vi "Read Message queue.vi"(8 "error in (no error)":errorcluster, 11 "Parent Actor in":refnum<class "Parent Actor.lvclass">) -> (0 "error out":errorcluster, 2 "Message queue":refnum<queue>, 3 "Parent Actor out":refnum<class "Parent Actor.lvclass">)   [LabVIEW 2015, in "Parent Actor.lvclass"]
uses:
  Parent Actor.lvclass
  Parent Message/Parent Message.lvclass
  Parent Actor.lvclass/Parent Actor.ctl
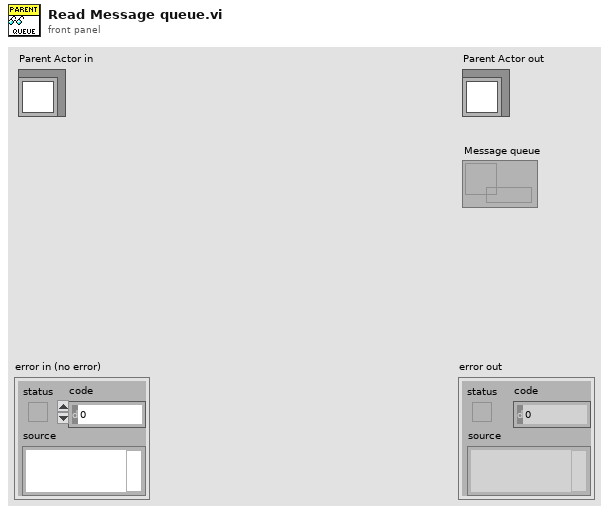
[diagram p1: front panel]
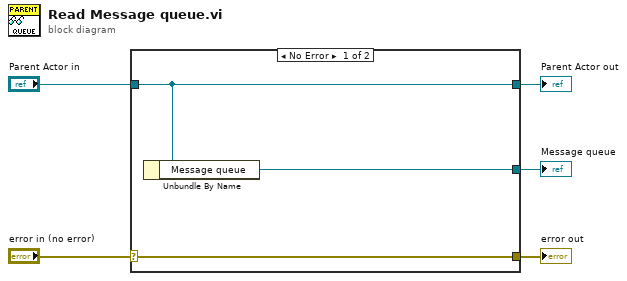
[diagram p0: block diagram]
diagram:
  n1 = case shown="No Error" "error in (no error)" {
    selector: "error in (no error)" -> [w8 w9]
    tunnel: [w8 w9] -> w4
    tunnel: [w7 w10] -> w2
    tunnel: "Parent Actor in" -> [w7 w10]
    tunnel: [w6 _] -> w1
    frame No Error {
      n2 = Unbundle By Name(w7) -> ("Message queue"=w6:refnum<queue>)
    }
    frame Error {
    }
  }
  "error out" <- w4
  "Parent Actor out" <- w2
  "Message queue" <- w1
